vi "DVR DeQ Loop.vi"(10 "DVR Q":refnum<data-value>) -> ()   [LabVIEW 2021, in "DVR Qs.lvlib"]
uses:
  DVR Qs.lvlib
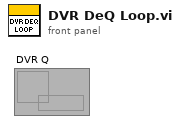
[diagram p1: front panel]
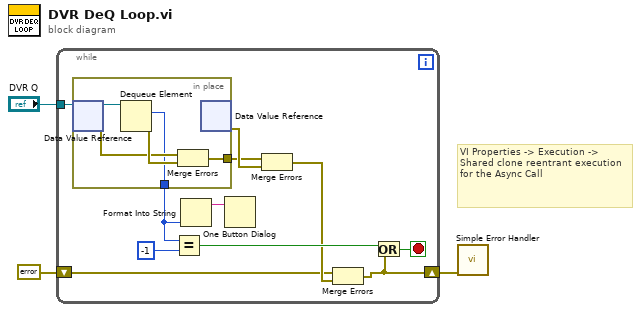
[diagram p0: block diagram]
diagram:
  # "VI Properties -> Execution -> Shared clone reentrant execution\nfor the Async Call"
  n1 = while {
    shift-right: [w10] -> w2
    shift-left: errorcluster {"status"=FALSE, "code"=0, "source"=""} ("error IO") -> [w4]
    tunnel: "DVR Q" -> [w9]
    stop <- w11 stop-if-true
    n2 = in-place {
      in-place-border: [w17] -> w7
      in-place-border: [w15] -> w6
      n3 = in-place-dvr #1(w9) -> (w19:refnum<queue>, w16:errorcluster)
      n4 = Dequeue Element(queue=w19) -> (element=w15:i32, error out=w18:errorcluster)  [unwired: 2 in, 2 out]
      n5 = Merge Errors(w16, w18) -> (w17:errorcluster)
      n6 = in-place-dvr #1() -> (w8:errorcluster)  [unwired: 1 in, 1 out]
    }
    n7 = Equal?(x=w6, y=-1) -> (x = y?=w14:bool)
    n8 = Format Into String(w6) -> (resulting string=w12:string)  [unwired: 3 in, 1 out]
    n9 = One Button Dialog(message=w12) -> ()  [unwired: 1 in, 1 out]
    n10 = Merge Errors(w7, w8) -> (w5:errorcluster)
    n11 = Merge Errors(w4, w5) -> (w10:errorcluster)
    n12 = Or(x=w14, y=w10) -> (x .or. y?=w11:bool)
  }
  n13 = call <vilib>:"Simple Error Handler.vi"("error in (no error)"=w2) -> ()  [unwired: 4 in, 5 out]
